vi "Plot Load maker V2 - scalewrite grid colors.vi"(8 "error in (no error)":errorcluster, 9 "Meta":T1, 10 "Scale reference":refnum<vi>, 11 "Meta LUT":refnum<data-value>) -> (0 "error out":errorcluster, 2 "Scale reference":refnum<vi>, 3 "Meta LUT":refnum<data-value>)   [LabVIEW 2021, in "RocketPlot.lvlib"]
uses:
  RocketPlot.lvlib
  TypeDefs/Plot scale meta JSON.ctl
  TypeDefs/Plot axis.ctl
  TypeDefs/Plot scale meta state.ctl
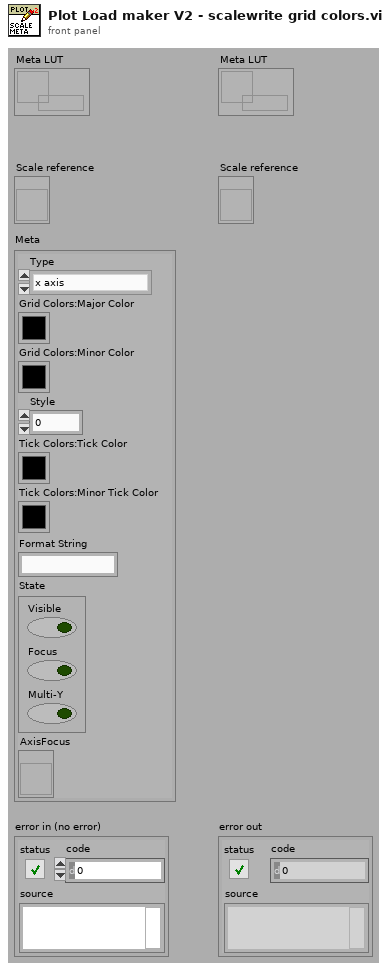
[diagram p1: front panel]
types:
  T1 = typedef "RocketPlot.lvlib/Plot scale meta JSON.ctl" = cluster{"Type":T2, "Grid Colors:Major Color":u32, "Grid Colors:Minor Color":u32, "Style":u8, "Tick Colors:Tick Color":u32, "Tick Colors:Minor Tick Color":u32, "Format String":string, "State":T3, "AxisFocus":refnum<vi>}
  T2 = typedef "RocketPlot.lvlib/Plot axis.ctl" = enum16{"x axis", "left axis", "right axis"}
  T3 = typedef "RocketPlot.lvlib/Plot scale meta state.ctl" = cluster{"Visible":bool, "Focus":bool, "Multi-Y":bool}
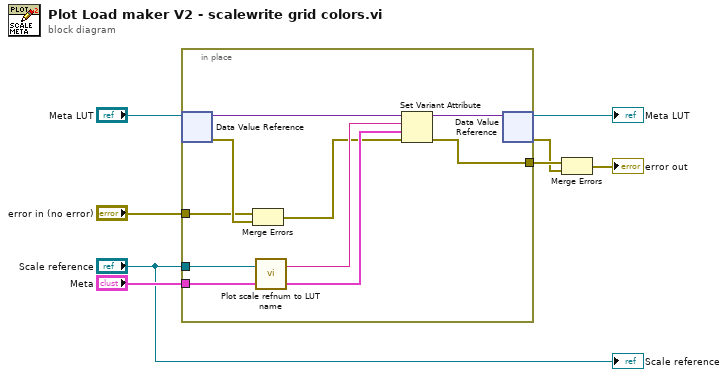
[diagram p0: block diagram]
diagram:
  n1 = in-place {
    in-place-border: "Meta" -> [w17]
    in-place-border: "Scale reference" -> [w16]
    in-place-border: "error in (no error)" -> [w11]
    in-place-border: [w9] -> w3
    n2 = in-place-dvr #1("Meta LUT") -> (w14:variant, w12:errorcluster)
    n3 = Merge Errors(w11, w12) -> (w10:errorcluster)
    n4 = call "Plot scale refnum to LUT name.vi"("Scale reference"=w16) -> ("scale reference variant lookup name"=w15:string)  [unwired: 2 in]
    n5 = Set Variant Attribute(Variant=w14, name=w15, value=w17, error in=w10) -> (Variant out=w13:variant, error out=w9:errorcluster)  [unwired: 1 out]
    n6 = in-place-dvr #1(w13) -> (→"Meta LUT":refnum<data-value>, w2:errorcluster)
  }
  n7 = Merge Errors(w3, w2) -> (→"error out":errorcluster)
  "Scale reference" <- "Scale reference"
